vi "Sistema de ventilación.vi"() -> ()   [LabVIEW 2023]
uses:
  <vilib>/MakerHub/LINX/LMH-LINX.lvlib
  <vilib>/MakerHub/LINX/Public/Sensors/Temperature/TMP3x/TMP3x.lvlib
  <vilib>/MakerHub/LINX/Public/Peripherals/Digital/Digital Write 1 Chan.vi
  <vilib>/MakerHub/LINX/Public/Peripherals/Analog/Analog Read 1 Chan.vi
  <vilib>/MakerHub/LINX/Public/Sensors/Temperature/TMP3x/TMP35.vi
  <vilib>/Instr/_visa.llb/VISA Configure Serial Port (Instr).vi
panel:
  out "Serevo Temp Angulo":string
  in  "VISA resource name":refnum<visa-resource-name>
  out "?":bool
  out "?":bool
  out "?":bool
  out "?":bool
  out "?":bool
  out "?":bool
  out "?":bool
  out "?":bool
  out "?":bool
  out "?":bool
  out "?":bool
  out "?":bool
  out "?":bool
  out "?":bool
  out "?":bool
  out "?":bool
  out "?":bool
  out "?":bool
  in  "Ventilador":bool
  out "Filtro de Calor":bool
  out "Filtro de Aire":bool
  out "?":dbl(knob) scale=0.0..1800.0
  out "Temperatura":dbl(slide) scale=0.0..60.0
  out "t [sec]":dbl
  out "Iteration No":i32
  in  "?":bool
  out "VI is running?":bool caption="ON/OFF"
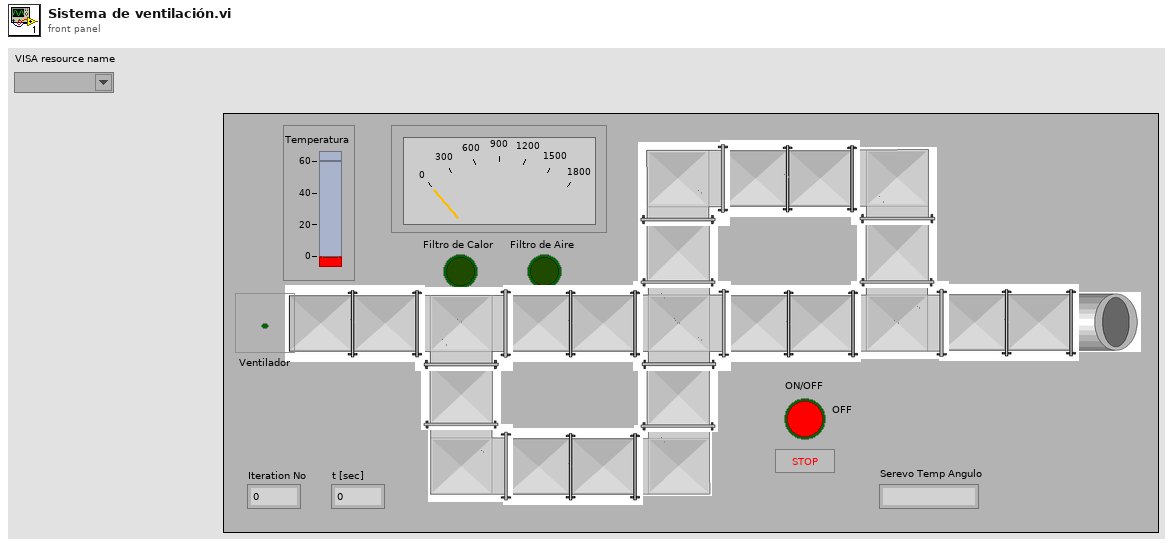
[diagram p1: front panel]
types:
  T1 = typedef "LMH-LINX.lvlib/LINX Ref.ctl" = cluster{"IO":T2, "Interface":T3, "LINX Device Config":T4}
  T2 = typedef "LMH-LINX.lvlib/Platform.ctl" = enum16{"Remote", "Local"}
  T3 = typedef "LMH-LINX.lvlib/Interface.ctl" = enum16{"Serial", "TCP"}
  T4 = typedef "LMH-LINX.lvlib/Device.lvlib/LINX Device Config.ctl" = cluster{"Interface":T3, "COM Port":refnum<visa-resource-name>, "TCP Configuration":T5, "Device Family":u8, "Device ID":u8, "Device Name":string, "TCP Ref":refnum<k5>, "Channels":T6}
  T5 = typedef "LMH-LINX.lvlib/Device.lvlib/TCP Config.ctl" = cluster{"IP Address":string, "Port":u16}
  T6 = typedef "LMH-LINX.lvlib/Channels.ctl" = cluster{"DI":u8[], "DO":u8[], "AI":u8[], "AO":u8[], "PWM":u8[], "QE":u8[], "UART":u8[], "I2C 2":u8[], "SPI":u8[], "CAN":u8[], "Servo":u8[], "AI Ref (V)":dbl, "AI Resolution (Bits)":u8, "AO Ref (V)":dbl, "AO Resolution (Bits)":u8}
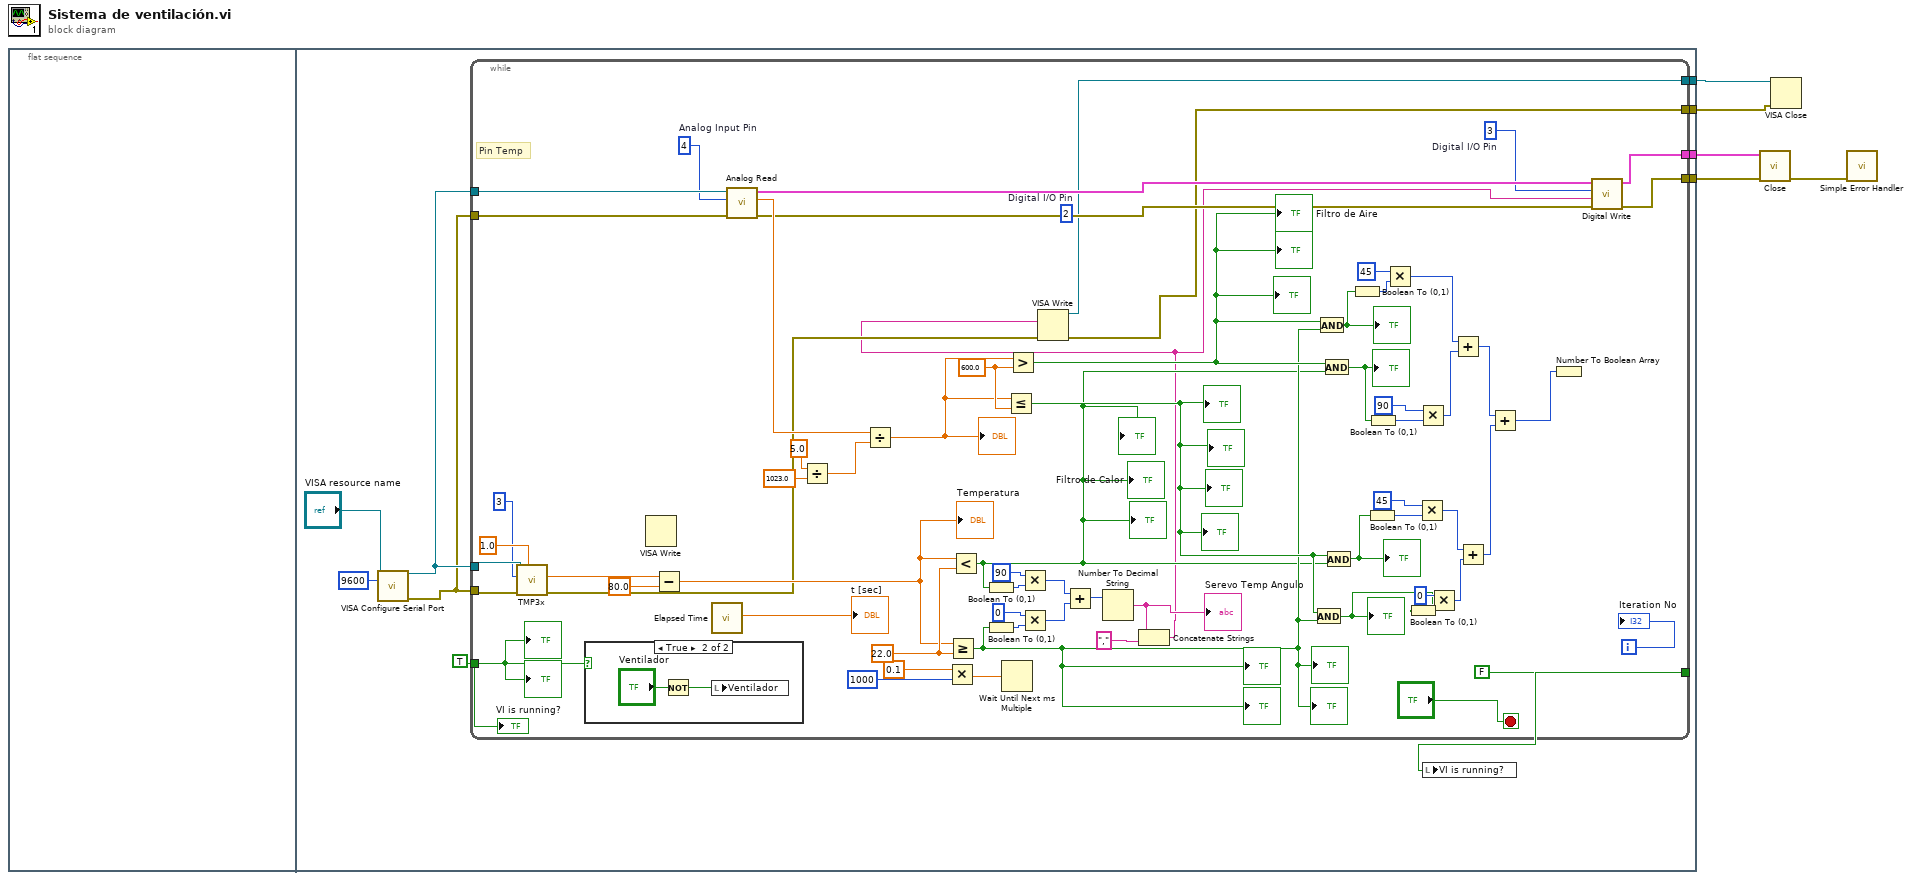
[diagram p0: block diagram]
diagram:
  n1 = flat-sequence {
    tunnel: [w13] -> w1
    tunnel: [w12] -> w4
    tunnel: [w11] -> w3
    tunnel: [w6] -> w2
    frame #0 {
    }
    frame #1 {
      n2 = call-poly "VISA Configure Serial Port"("VISA resource name"="VISA resource name", "baud rate (9600)"=u32 9600) -> ("VISA resource name out"=w8:refnum<visa-resource-name>, "error out"=w7:errorcluster)  [unwired: 12 in]
      n3 = while {
        tunnel: [FALSE] -> w14
        tunnel: TRUE -> [w75]
        tunnel: w8 -> [w74]
        tunnel: w7 -> [w72]
        tunnel: w8 -> [w67]
        tunnel: [w22] -> w13
        tunnel: w7 -> [w61]
        tunnel: [w56] -> w12
        tunnel: [w59] -> w11
        tunnel: [w21] -> w6
        i -> [w79]
        stop <- "?" stop-if-true
        w51 = 2  # Digital I/O Pin
        w55 = 3  # Digital I/O Pin
        w60 = 4  # Analog Input Pin
        w77 = 600.0
        w76 = 22.0
        # "Pin Temp"
        n4 = call-poly <vilib>:"TMP3x.vi"("Analog Ref Override"=1.0, "Error In"=w72, "Analog Channel"=3, "LINX Resource"=w74) -> ("Error Out"=w23:errorcluster, "Temp C"=w70:dbl, "LINX Resource"=w52:T1)  [unwired: 5 in]
        n5 = case shown="True" w75 {
          frame False {
          }
          frame True {
            n6 = Not(x="Ventilador") -> (.not. x?=w85:bool)
            n7 = local write "Ventilador"(w85) -> ()
          }
        }
        n8 = VISA Write() -> ()  [unwired: 3 in, 3 out]
        n9 = Subtract(x=w70, y=80.0) -> (x-y=w69:dbl)
        "Temperatura" <- w69
        n10 = call "Elapsed Time"() -> ("Elapsed Time (s)"=→"t [sec]":dbl)  [unwired: 12 in, 7 out]
        n11 = call-poly <vilib>:"Analog Read.vi"("Error In"=w61, "Analog Channel"=w60, "LINX Resource"=w67) -> ("Error Out"=w58:errorcluster, "Voltage"=w64:dbl, "LINX Resource"=w57:T1)  [unwired: 5 in, 1 out]
        n12 = Divide(x=5.0, y=1023.0) -> (x/y=w63:dbl)
        n13 = Divide(x=w64, y=w63) -> (x/y=w62:dbl)
        "?" <- w62
        n14 = Multiply(x=0.1, y=1000) -> (x*y=w82:dbl)
        n15 = Greater Or Equal?(x=w69, y=w76) -> (x >= y?=w27:bool)
        "?" <- w27
        "?" <- w27
        "?" <- w27
        "?" <- w27
        n16 = Less?(x=w69, y=w76) -> (x < y?=w26:bool)
        "Filtro de Calor" <- w26
        "?" <- w26
        "?" <- w26
        n17 = Boolean To (0,1)(Boolean=w26) -> (0, 1=w30:i16)
        n18 = Boolean To (0,1)(Boolean=w27) -> (0, 1=w28:i16)
        n19 = Wait Until Next ms Multiple(millisecond multiple=w82) -> ()  [unwired: 1 out]
        n20 = Less Or Equal?(x=w62, y=w77) -> (x <= y?=w68:bool)
        "?" <- w68
        "?" <- w68
        "?" <- w68
        "?" <- w68
        n21 = Greater?(x=w62, y=w77) -> (0:w54:bool)
        "Filtro de Aire" <- w54
        "?" <- w54
        "?" <- w54
        n22 = Multiply(x=90, y=w30) -> (x*y=w24:i32)
        n23 = Multiply(x=0, y=w28) -> (x*y=w25:i32)
        n24 = Add(x=w24, y=w25) -> (x+y=w20:i32)
        n25 = Number To Decimal String(number=w20) -> (decimal integer string=w19:string)  [unwired: 1 in]
        "Serevo Temp Angulo" <- w19
        n26 = Concatenate Strings(w19, "," ("string")) -> (w17:string)
        n27 = VISA Write(write buffer=w17, error in (no error)=w23) -> (VISA resource name out=w21:refnum<visa-resource-name>, error out=w22:errorcluster)  [unwired: 1 in, 1 out]
        n28 = And(x=w68, y=w27) -> (x .and. y?=w42:bool)
        "?" <- w42
        n29 = And(x=w54, y=w27) -> (x .and. y?=w49:bool)
        "?" <- w49
        n30 = And(x=w54, y=w26) -> (x .and. y?=w39:bool)
        "?" <- w39
        n31 = And(x=w68, y=w26) -> (x .and. y?=w45:bool)
        "?" <- w45
        n32 = Boolean To (0,1)(Boolean=w49) -> (0, 1=w48:i16)
        n33 = Boolean To (0,1)(Boolean=w45) -> (0, 1=w46:i16)
        n34 = Boolean To (0,1)(Boolean=w39) -> (0, 1=w40:i16)
        n35 = Multiply(x=45, y=w48) -> (x*y=w38:i32)
        n36 = Boolean To (0,1)(Boolean=w42) -> (0, 1=w43:i16)
        n37 = Multiply(x=45, y=w46) -> (x*y=w35:i32)
        n38 = Multiply(x=90, y=w40) -> (x*y=w37:i32)
        n39 = Multiply(x=0, y=w43) -> (x*y=w36:i32)
        n40 = Add(x=w38, y=w37) -> (x+y=w33:i32)
        n41 = Add(x=w35, y=w36) -> (x+y=w34:i32)
        n42 = Add(x=w33, y=w34) -> (x+y=w32:i32)
        n43 = Number To Boolean Array(number=w32) -> (Boolean array=w16:bool[])
        n44 = call-poly <vilib>:"Digital Write.vi"("Error In"=w58, "Output Value"=w17, "DO Channel"=w55, "LINX Resource"=w57) -> ("Error Out"=w59:errorcluster, "LINX Resource"=w56:T1)  [unwired: 6 in]
        "VI is running?" <- w75
        "Iteration No" <- w79
        "?" <- w75
        "?" <- w75
      }
      n45 = local write "VI is running?"(w14) -> ()
    }
  }
  n46 = call <vilib>:"Close.vi"("Error In"=w3, "LINX Resource"=w4) -> ("Error Out"=w5:errorcluster)  [unwired: 9 in]
  n47 = VISA Close(VISA resource name=w2, error in (no error)=w1) -> ()  [unwired: 1 out]
  n48 = call <vilib>:"Simple Error Handler.vi"("error in (no error)"=w5) -> ()  [unwired: 4 in, 5 out]
